vi "Config Cameras.vi"(8 "error in (no error)":errorcluster, 11 "FlexWorktable in":refnum<class "FlexWorktable.lvclass">) -> (0 "error out":errorcluster, 2 "Array":string[](array[string]), 3 "FlexWorktable out":refnum<class "FlexWorktable.lvclass">)   [LabVIEW 2017, in "FlexWorktable.lvclass"]
uses:
  FlexWorktable.lvclass
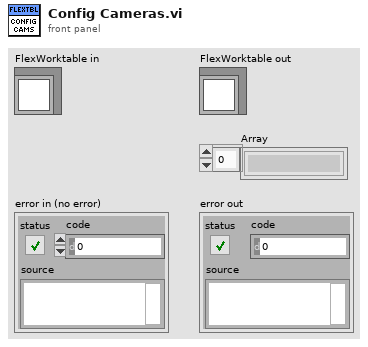
[diagram p1: front panel]
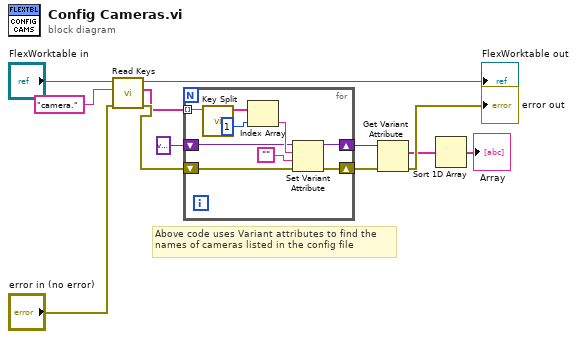
[diagram p0: block diagram]
diagram:
  # "Above code uses Variant attributes to find the\nnames of cameras listed in the config file"
  n1 = call-dynamic "Read Keys.vi"("error in (no error)"="error in (no error)", "Selector"="camera.", "FlexWorktable in"="FlexWorktable in") -> ("error out"=w7:errorcluster, "Keys"=w4:string[], "FlexWorktable out"=→"FlexWorktable out":refnum<class "FlexWorktable.lvclass">)  [unwired: 6 in]
  n2 = for {
    tunnel: w4 -> [w21] mode=indexing
    shift-right: [w16] -> w6
    shift-left: variant -> [w17]
    shift-right: [w13] -> w8
    shift-left: w7 -> [w14]
    n3 = call "Key Split.vi"("Key"=w21) -> ("Key Elements"=w20:string[])  [unwired: 10 in]
    n4 = Index Array(array=w20, index=1) -> (element=w18:string)
    n5 = Set Variant Attribute(Variant=w17, name=w18, value="", error in=w14) -> (Variant out=w16:variant, error out=w13:errorcluster)  [unwired: 1 out]
  }
  n6 = Get Variant Attribute(Variant=w6, error in=w8) -> (names=w9:string[], error out=→"error out":errorcluster)  [unwired: 2 in, 2 out]
  n7 = Sort 1D Array(array=w9) -> (sorted array=→"Array":string[])
